vi "myRIO_Init.vi"(8 "error in":errorcluster) -> (0 "error out":errorcluster, 2 "AI Ref Out":T1, 3 "I2C Ref Out":T10)   [LabVIEW 2019]
uses:
  <vilib>/myRIO/Instrument Drivers/Onboard IO/I2C/typedefs/I2C Reference.ctl
  <vilib>/myRIO/Common/Instrument Driver Framework/Utilities/typedefs/myRIO Generic Hardware Reference.ctl
  <vilib>/myRIO/Common/Instrument Driver Framework/Utilities/typedefs/Hardware Version Enum.ctl
  <vilib>/myRIO/Common/Instrument Driver Framework/Utilities/typedefs/myRIO v1.0 Reference.ctl
  <vilib>/myRIO/Common/Instrument Driver Framework/Utilities/typedefs/Generic FPGA Reference.ctl
  <vilib>/myRIO/Common/Instrument Driver Framework/myRIO v1.0/I2C/typedefs/I2C Channels Enum.ctl
  <vilib>/myRIO/Instrument Drivers/Onboard IO/I2C/typedefs/I2C Configuration.ctl
  <vilib>/myRIO/Instrument Drivers/Onboard IO/I2C/typedefs/I2C Transfer Rate.ctl
  <vilib>/myRIO/Instrument Drivers/Onboard IO/AI/typedefs/AI Reference.ctl
  <vilib>/myRIO/Common/Instrument Driver Framework/myRIO v1.0/AI/typedefs/AI Channels List.ctl
  <vilib>/myRIO/Common/Instrument Driver Framework/myRIO v1.0/AI/typedefs/AI Channels Enum.ctl
  <vilib>/myRIO/Common/Instrument Driver Framework/Utilities/typedefs/Analog Scaling Constants List.ctl
  <vilib>/myRIO/Common/Instrument Driver Framework/Utilities/typedefs/Analog Scaling Constants.ctl
  TypeDef/#TypeDef_EnumSensorConnection.ctl
  <vilib>/userdefined/High Color/nirio_resource_hc.ctl
  <vilib>/myRIO/Common/Instrument Driver Framework/myRIO v1.0/AI/vis/myRIO v1.1 Open AI.vi
  <vilib>/myRIO/Common/Instrument Driver Framework/myRIO v1.0/I2C/vis/myRIO v1.1 Open I2C.vi
  <vilib>/myRIO/Common/Instrument Driver Framework/Utilities/vis/Validate Channels.vi
  <vilib>/myRIO/Common/Instrument Driver Framework/myRIO v1.0/AI/vis/myRIO v1.0 Reserve AI.vi
  <vilib>/myRIO/Common/Instrument Driver Framework/myRIO v1.0/I2C/vis/myRIO v1.0 Reserve I2C.vi
  <vilib>/myRIO/Common/Instrument Driver Framework/myRIO v1.0/AI/vis/myRIO v1.0 Build MUX Configuration AI.vi
  <vilib>/myRIO/Common/Instrument Driver Framework/myRIO v1.0/Resource Manager/vis/myRIO v1.0 Reserve Channel List.vi
  <vilib>/myRIO/Common/Instrument Driver Framework/myRIO v1.0/I2C/vis/myRIO v1.0 Build MUX Configuration I2C.vi
  <vilib>/myRIO/Common/Instrument Driver Framework/myRIO v1.0/Resource Manager/vis/myRIO v1.0 Reserve Channel.vi
  <vilib>/myRIO/Common/Instrument Driver Framework/myRIO v1.0/Resource Manager/vis/myRIO v1.0 Unreserve Channel.vi
  <vilib>/myRIO/Common/Instrument Driver Framework/myRIO v1.0/Resource Manager/vis/myRIO v1.0 Create Configuration List.vi
  <vilib>/myRIO/Common/Instrument Driver Framework/myRIO v1.0/Resource Manager/vis/myRIO v1.0 Build Mutex Name.vi
  <vilib>/Utility/VariantDataType/GetNumericInfo.vi
  <vilib>/Utility/error.llb/Error Cluster From Error Code.vi
  <vilib>/myRIO/Common/Instrument Driver Framework/myRIO v1.0/myRIO v1.1 Open.vi
  <vilib>/myRIO/Common/Instrument Driver Framework/myRIO v1.0/AI/vis/myRIO v1.0 Get Scaling Constants AI.vi
  <vilib>/myRIO/Common/Instrument Driver Framework/Utilities/vis/IO Manager.vi
  <vilib>/myRIO/Common/Instrument Driver Framework/Utilities/vis/Configuration Manager.vi
  <vilib>/myRIO/Common/Instrument Driver Framework/myRIO v1.0/myRIO v1.0 Close.vi
  <vilib>/myRIO/Common/Instrument Driver Framework/myRIO v1.0/Resource Manager/vis/myRIO v1.0 Configure IO.vi
  <vilib>/myRIO/Common/Instrument Driver Framework/myRIO v1.0/I2C/vis/myRIO v1.0 Configure I2C.vi
  <vilib>/myRIO/Common/Instrument Driver Framework/myRIO v1.0/I2C/vis/myRIO v1.0 Write I2C.vi
  <vilib>/myRIO/Common/Instrument Driver Framework/myRIO v1.0/I2C/vis/myRIO v1.0 Read I2C.vi
  <vilib>/myRIO/Instrument Drivers/Onboard IO/AI/vis/myRIO AI Open.xnode
  <vilib>/myRIO/Instrument Drivers/Onboard IO/I2C/typedefs/I2C User Configuration.ctl
  <vilib>/myRIO/Instrument Drivers/Onboard IO/I2C/vis/myRIO I2C Open.xnode
  <vilib>/myRIO/Instrument Drivers/Onboard IO/I2C/I2C.lvlib
  <vilib>/myRIO/Instrument Drivers/Onboard IO/AI/AI.lvlib
panel:
  out "1/x":dbl
  out "Offset (Volts)":dbl
  out "LSB Weight (Volts)":dbl
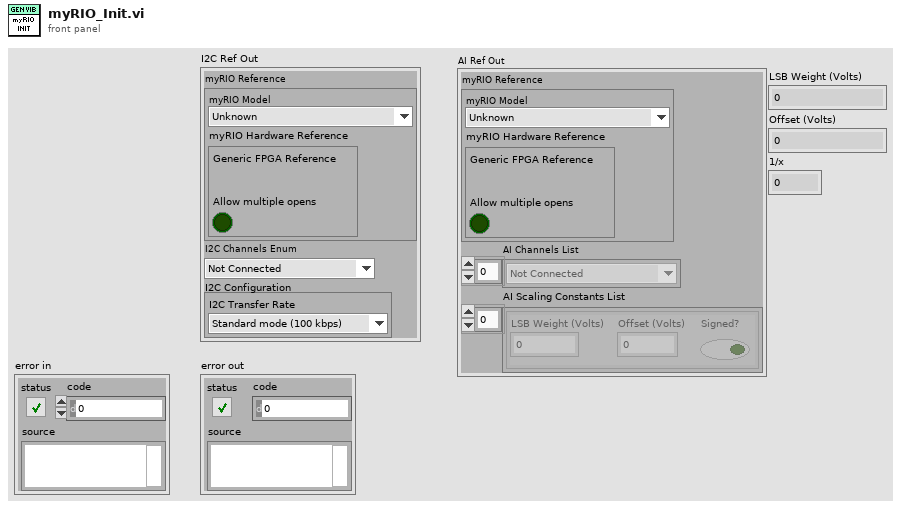
[diagram p1: front panel]
types:
  T1 = typedef "AI.lvlib/AI Reference.ctl" = cluster{"myRIO Reference":T2, "AI Channels List":T6, "AI Scaling Constants List":T8}
  T2 = typedef "myRIO Generic Hardware Reference.ctl" = cluster{"myRIO Model":T3, "myRIO Hardware Reference":T4}
  T3 = typedef "Hardware Version Enum.ctl" = enum16{"Unknown", "myRIO-1900", "myRIO-1950", "roboRIO", "NI ELVIS RIO CM", "ELVIS III"}
  T4 = typedef "myRIO v1.0 Reference.ctl" = cluster{"Generic FPGA Reference":T5, "Allow multiple opens":bool}
  T5 = typedef "Generic FPGA Reference.ctl" = refnum<k20>
  T6 = typedef "AI Channels List.ctl" = T7[]
  T7 = typedef "AI Channels Enum.ctl" = enum16{"Not Connected", "AudioIn/Left", "AudioIn/Right", "C/AI0", "C/AI1", "A/AI0", "A/AI1", "A/AI2", "A/AI3", "A/AI4", "A/AI5", "A/AI6", "A/AI7", "B/AI0", "B/AI1", "B/AI2", "B/AI3", "B/AI4", "B/AI5", "B/AI6", "B/AI7", "AI/AI0", "AI/AI1", "AI/AI2", "AI/AI3", "A/AI0 (DIFF)", "A/AI1 (DIFF)", "A/AI2 (DIFF)", "A/AI3 (DIFF)", "B/AI0 (DIFF)", "B/AI1 (DIFF)", "B/AI2 (DIFF)", "B/AI3 (DIFF)"}
  T8 = typedef "Analog Scaling Constants List.ctl" = T9[]
  T9 = typedef "Analog Scaling Constants.ctl" = cluster{"LSB Weight (Volts)":dbl, "Offset (Volts)":dbl, "Signed?":bool}
  T10 = typedef "I2C.lvlib/I2C Reference.ctl" = cluster{"myRIO Reference":T2, "I2C Channels Enum":T11, "I2C Configuration":T12}
  T11 = typedef "I2C Channels Enum.ctl" = enum16{"Not Connected", "A/I2C", "B/I2C", "I2C/I2C"}
  T12 = typedef "I2C.lvlib/I2C Configuration.ctl" = cluster{"I2C Transfer Rate":T13}
  T13 = typedef "I2C.lvlib/I2C Transfer Rate.ctl" = enum16{"Standard mode (100 kbps)", "Fast mode (400 kbps)"}
  T14 = typedef "#TypeDef_EnumSensorConnection.ctl" = enum16{"Analog", "Digital"}
  T15 = typedef "nirio_resource_hc.ctl" = tag
  T16 = typedef "I2C.lvlib/I2C User Configuration.ctl" = cluster{"I2C Transfer Rate":T13}
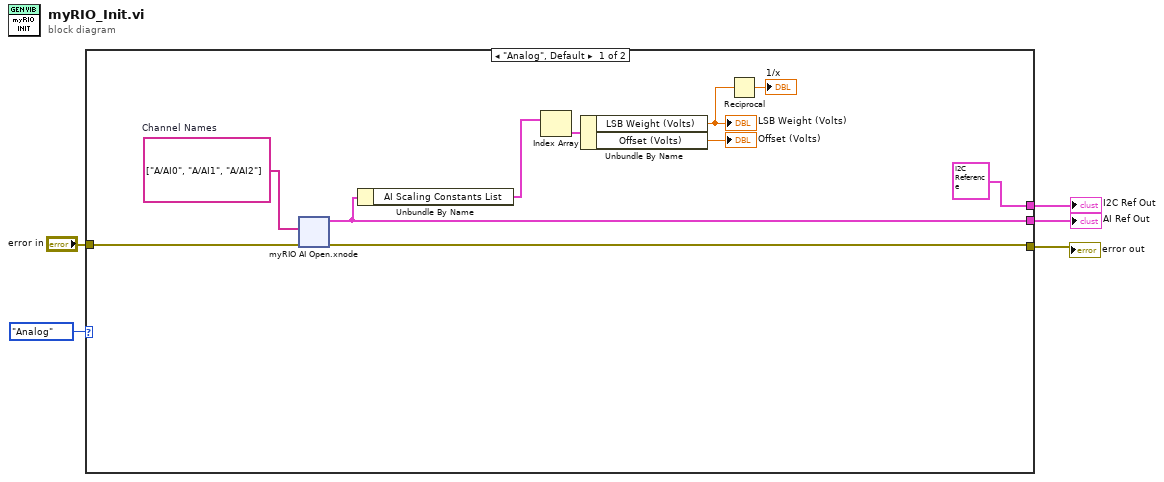
[diagram p0: block diagram]
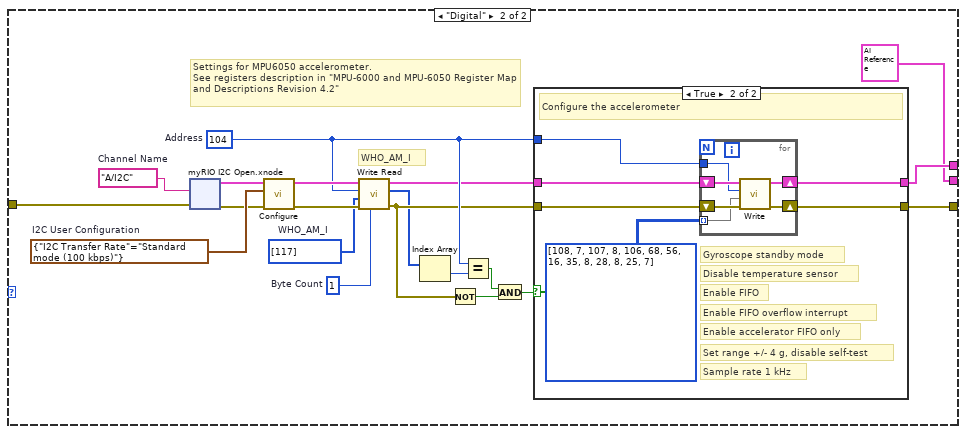
[diagram p2: hidden frame]
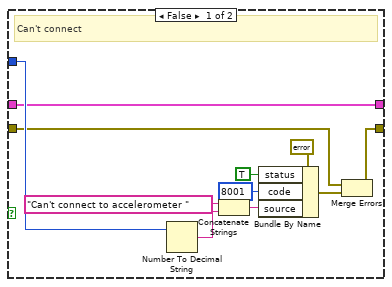
[diagram p3: hidden frame]
diagram:
  n1 = case shown="\"Analog\", Default" #TypeDef_EnumSensorConnection."Analog" {
    tunnel: [w14 w53] -> w5
    tunnel: [T10 {"myRIO Reference"={"myRIO Model"=enum."Unknown", "myRIO Hardware Reference"={"Generic FPGA Reference"=refnum, "Allow multiple opens"=FALSE}}, "I2C Channels Enum"=enum."Not Connected", "I2C Configuration"={"I2C Transfer Rate"=enum."Standard mode (100 kbps)"}} ("I2C Ref Out") w46] -> w3
    tunnel: "error in" -> [w15 w35]
    tunnel: [w11 T1 {"myRIO Reference"={"myRIO Model"=enum."Unknown", "myRIO Hardware Reference"={"Generic FPGA Reference"=refnum, "Allow multiple opens"=FALSE}}, "AI Channels List"=[], "AI Scaling Constants List"=[]} ("AI Ref Out")] -> w2
    frame "Analog", Default {
      w12 = tag[] ["A/AI0", "A/AI1", "A/AI2"]  # Channel Names
      n2 = xnode "myRIO AI Open.xnode"("error in (no error)"=w15, "Channel Names"=w12) -> ("error out"=w14:errorcluster, "AI Ref Out"=w11:T1)  [unwired: 1 in]
      n3 = Unbundle By Name(w11) -> ("AI Scaling Constants List"=w10:T8)
      n4 = Index Array(array=w10) -> (element=w8:T9)  [unwired: 1 in]
      n5 = Unbundle By Name(w8) -> ("LSB Weight (Volts)"=w7:dbl, "Offset (Volts)"=→"Offset (Volts)":dbl)
      "LSB Weight (Volts)" <- w7
      n6 = Reciprocal(x=w7) -> (1/x=→"1/x":dbl)
    }
    frame "Digital" {
      w52 = T16 {"I2C Transfer Rate"=enum."Standard mode (100 kbps)"}  # I2C User Configuration
      w47 = tag "A/I2C"  # Channel Name
      w44 = u8 104  # Address
      w38 = u32 1  # Byte Count
      w39 = u8[] [117]  # WHO_AM_I
      # "Settings for MPU6050 accelerometer.\nSee registers description in \"MPU-6000 and MPU-6050 Register Map and Descriptions Revision 4.2\""
      # "WHO_AM_I"
      n7 = xnode "myRIO I2C Open.xnode"("error in (no error)"=w35, "Channel Name"=w47) -> ("error out"=w49:errorcluster, "I2C Ref Out"=w48:T10)  [unwired: 1 in]
      n8 = call <vilib>:"Configure.vi"("error in (no error)"=w49, "I2C User Configuration"=w52, "I2C Ref In"=w48) -> ("error out"=w51:errorcluster, "I2C Ref Out"=w50:T10)  [unwired: 7 in]
      n9 = call <vilib>:"Write Read.vi"("Byte Count"=w38, "error in (no error)"=w51, "Bytes to Write"=w39, "Slave Address (7-bit)"=w44, "I2C Ref In"=w50) -> ("error out"=w42:errorcluster, "Bytes Read"=w37:u8[], "I2C Ref Out"=w40:T10)  [unwired: 3 in]
      n10 = Index Array(array=w37) -> (element=w36:u8)  [unwired: 1 in]
      n11 = Not(x=w42) -> (.not. x?=w43:bool)
      n12 = Equal?(x=w44, y=w36) -> (x = y?=w41:bool)
      n13 = And(x=w41, y=w43) -> (x .and. y?=w45:bool)
      n14 = case shown="True" w45 {
        tunnel: w44 -> [w78 w83]
        tunnel: w40 -> [w71 w86]
        tunnel: w42 -> [w73 w85]
        tunnel: [w70 w82] -> w53
        tunnel: [w71 w81] -> w46
        frame False {
          # "Can't connect"
          n15 = Number To Decimal String(number=w78) -> (decimal integer string=w75:string)  [unwired: 1 in]
          n16 = Concatenate Strings("Can't connect to accelerometer " ("source"), w75) -> (w77:string)
          n17 = Bundle By Name(cluster=errorcluster {"status"=FALSE, "code"=0, "source"=""} ("error constant"), "status"=TRUE, "code"=8001, "source"=w77) -> (w72:errorcluster)
          n18 = Merge Errors(w73, w72) -> (w70:errorcluster)
        }
        frame True {
          # "Sample rate 1 kHz"
          # "Enable accelerator FIFO only"
          # "Disable temperature sensor"
          # "Gyroscope standby mode"
          # "Set range +/- 4 g, disable self-test"
          # "Enable FIFO"
          # "Enable FIFO overflow interrupt"
          # "Configure the accelerometer"
          n19 = for {
            shift-right: [w89] -> w82
            shift-left: w85 -> [w92]
            shift-right: [w90] -> w81
            shift-left: w86 -> [w91]
            tunnel: u8[][] [[108, 7], [107, 8], [106, 68], [56, 16], [35, 8], [28, 8], [25, 7]] ("Bytes to Write") -> [w88] mode=indexing
            tunnel: w83 -> [w87]
            n20 = call <vilib>:"Write.vi"("error in (no error)"=w92, "Bytes to Write"=w88, "Slave Address (7-bit)"=w87, "I2C Ref In"=w91) -> ("error out"=w89:errorcluster, "I2C Ref Out"=w90:T10)  [unwired: 6 in]
          }
        }
      }
    }
  }
  "error out" <- w5
  "I2C Ref Out" <- w3
  "AI Ref Out" <- w2
